vi "Resize hist cluster rolling array.vi"(8 "error in (no error)":errorcluster, 9 "Enum":T2(ring), 10 "Max number of elements":i32, 11 "Cluster":T1) -> (0 "error out":errorcluster)   [LabVIEW 2016]
uses:
  Typedefs/Coincidence histogram cluster refnum.ctl
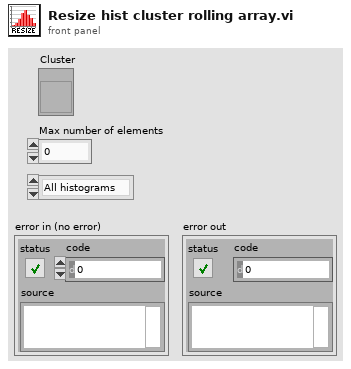
[diagram p1: front panel]
types:
  T1 = typedef "Coincidence histogram cluster refnum.ctl" = refnum<vi>
  T2 = enum16{"All histograms", "0x4", "0x5", "0x6", "0x7", "1x4", "1x5", "1x6", "1x7", "2x4", "2x5", "2x6", "2x7", "3x4", "3x5", "3x6", "3x7", "8x12", "8x13", "8x14", "8x15", "9x12", "9x13", "9x14", "9x15", "10x12", "10x13", "10x14", "10x15", "11x12", "11x13", "11x14", "11x15"}
  T3 = typedef "Coincidence single histogram.ctl" = cluster{"Histogram Graph":cluster{"X Values":dbl[], "Histogram: h(x)":i32[]}[], "IDs":i8[], "Datapoints:":i32, "S:":dbl, "Data array":cluster{"Data":i32[], "Max index":i32, "Current index":i32, "Numofpoints":i32}}
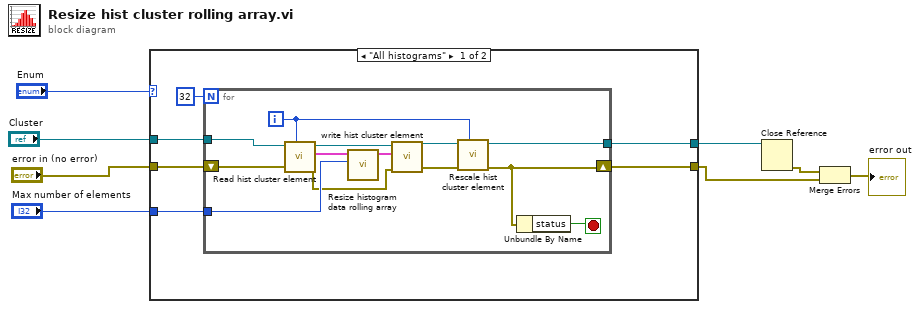
[diagram p0: block diagram]
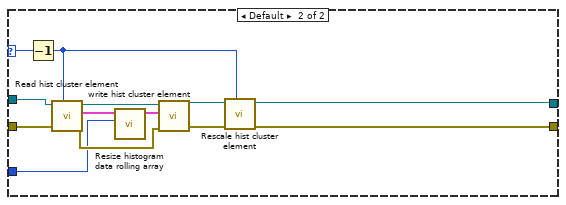
[diagram p2: hidden frame]
diagram:
  n1 = case shown="\"All histograms\"" "Enum" {
    selector: "Enum" -> [_ w32]
    tunnel: "error in (no error)" -> [w14 w34]
    tunnel: "Cluster" -> [w13 w31]
    tunnel: "Max number of elements" -> [w11 w33]
    tunnel: [w10 w28] -> w4
    tunnel: [w9 w29] -> w2
    frame "All histograms" {
      n2 = for {
        N: 32 -> [_]
        tunnel: w13 -> [w26]
        shift-right: [w17] -> w9
        shift-left: w14 -> [w27]
        tunnel: w11 -> [w24]
        tunnel: [w15] -> w10
        i -> [w18]
        stop <- w16 stop-if-true
        n3 = call "Read hist cluster element.vi"("Hist cluster element"=w18, "error in (no error)"=w27, "histogram in"=w26) -> ("error out"=w22:errorcluster, "histogram"=w25:T3, "histogram out"=w23:T1)  [unwired: 6 in]
        n4 = call "Resize histogram data rolling array.vi"("New max size"=w24, "histogram"=w25) -> ("output cluster"=w21:T3)  [unwired: 9 in]
        n5 = call "write hist cluster element.vi"("error in (no error)"=w22, "histogram"=w21, "Hist cluster"=w23) -> ("error out"=w19:errorcluster, "Hist cluster"=w20:T1)  [unwired: 7 in]
        n6 = call "Rescale hist cluster element.vi"("Hist cluster element"=w18, "error in (no error)"=w19, "Hist cluster"=w20) -> ("error out"=w17:errorcluster, "Hist cluster"=w15:T1)  [unwired: 7 in]
        n7 = Unbundle By Name(w17) -> ("status"=w16:bool)
      }
    }
    frame Default {
      n8 = Decrement(x=w32) -> (x-1=w30:T2)
      n9 = call "Read hist cluster element.vi"("Hist cluster element"=w30, "error in (no error)"=w34, "histogram in"=w31) -> ("error out"=w38:errorcluster, "histogram"=w40:T3, "histogram out"=w39:T1)  [unwired: 6 in]
      n10 = call "Resize histogram data rolling array.vi"("New max size"=w33, "histogram"=w40) -> ("output cluster"=w37:T3)  [unwired: 9 in]
      n11 = call "write hist cluster element.vi"("error in (no error)"=w38, "histogram"=w37, "Hist cluster"=w39) -> ("error out"=w35:errorcluster, "Hist cluster"=w36:T1)  [unwired: 7 in]
      n12 = call "Rescale hist cluster element.vi"("Hist cluster element"=w30, "error in (no error)"=w35, "Hist cluster"=w36) -> ("error out"=w29:errorcluster, "Hist cluster"=w28:T1)  [unwired: 7 in]
    }
  }
  n13 = Close Reference(reference=w4) -> (error out=w3:errorcluster)  [unwired: 1 in]
  n14 = Merge Errors(w3, w2) -> (→"error out":errorcluster)
